vi "LWXPS_PositionerCompensationPhaseCorrectionFiltersSet.vi"(0 "Numerator Frequency 1":dbl, 1 "Positioner Name":string, 2 "XPS Reference IN":refnum<k24>, 5 "Denominator Frequency 1":dbl, 7 "Phase Correction Gain 1":dbl, 9 "Numerator Frequency 2":dbl, 11 "Denominator Frequency 2":dbl, 12 "Phase Correction Gain 2":dbl, 13 "LabVIEW error IN":errorcluster) -> (4 "XPS Reference OUT":refnum<k24>, 6 "Returned error code":i32, 8 "XPS Error String":string, 15 "LabVIEW error OUT":errorcluster)   [LabVIEW 2014]
uses:
  D:/XPSQ8_LabView_Library/Development/Source/Dll/Newport.XPS.CommandInterface.dll
  Dll/Newport.XPS.CommandInterface.dll
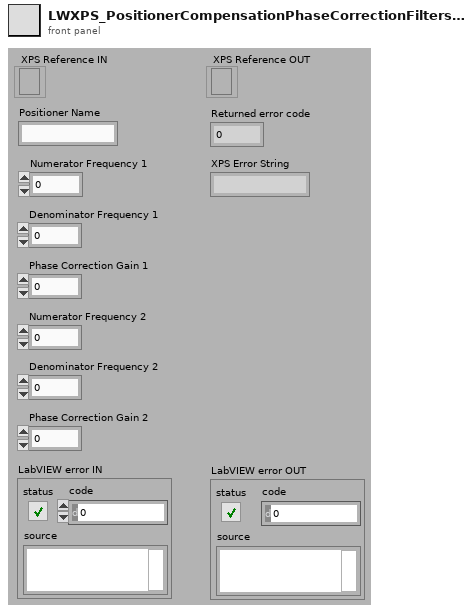
[diagram p1: front panel]
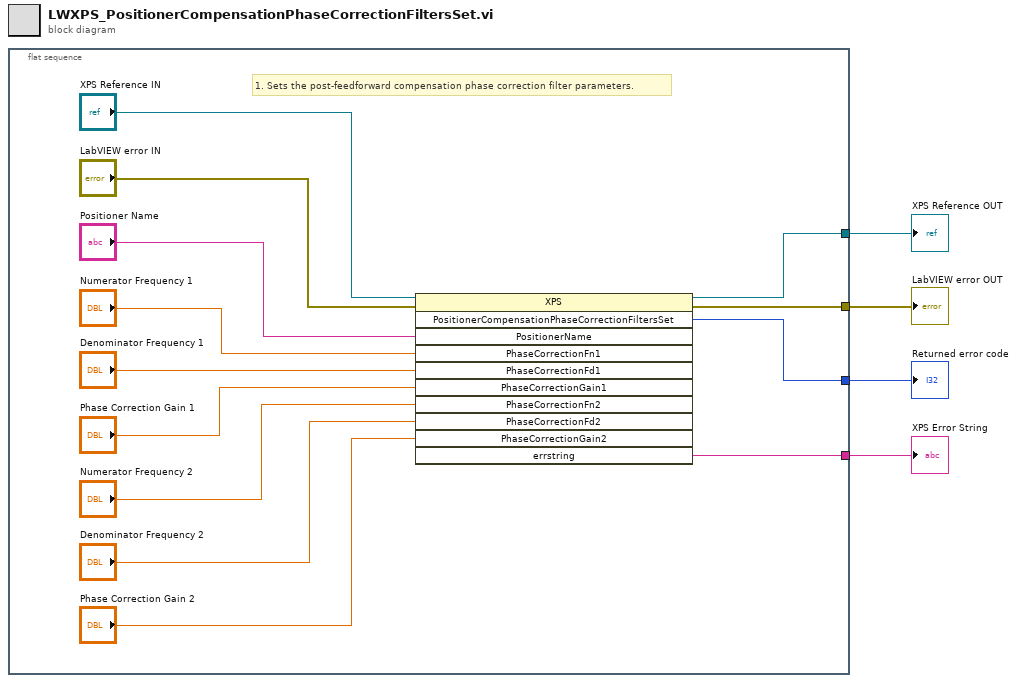
[diagram p0: block diagram]
diagram:
  n1 = flat-sequence {
    tunnel: [w13] -> w4
    tunnel: [w12] -> w3
    tunnel: [w14] -> w2
    tunnel: [w5] -> w1
    frame #0 {
      # "1. Sets the post-feedforward compensation phase correction filter parameters."
      n2 = invoke class="XPS" method="PositionerCompensationPhaseCorrectionFiltersSet"(reference="XPS Reference IN", error in="LabVIEW error IN", "PositionerName"="Positioner Name", "PhaseCorrectionFn1"="Numerator Frequency 1", "PhaseCorrectionFd1"="Denominator Frequency 1", "PhaseCorrectionGain1"="Phase Correction Gain 1", "PhaseCorrectionFn2"="Numerator Frequency 2", "PhaseCorrectionFd2"="Denominator Frequency 2", "PhaseCorrectionGain2"="Phase Correction Gain 2") -> (reference out=w13:refnum<k24>, error out=w12:errorcluster, "PositionerCompensationPhaseCorrectionFiltersSet"=w14:i32, "errstring"=w5:string)  [unwired: 2 in, 7 out]
    }
  }
  "XPS Error String" <- w1
  "XPS Reference OUT" <- w4
  "LabVIEW error OUT" <- w3
  "Returned error code" <- w2
